vi "gloablDefinitions.vi"() -> ()   [LabVIEW 2017]
panel:
  in  "Matlab Lib Path":path=path "C:/Code/CMCryoSysCode/Matlab"
  in  "Template Search Path":path=path "C:/Code/CMCryoSysLabView/Experiments"
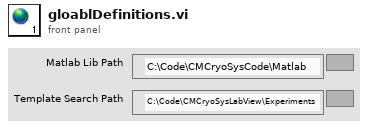
[diagram p1: front panel]
diagram:
